vi "Configure Sampling.vi"(0 "VISA resource in":refnum<visa-resource-name>, 1 "sample period [s] (-1: use EXT trig as source)":dbl=-1.0 format="%#_6p", 2 "apperture [s] (1.4us)":dbl=1.4e-06 format="%#_6p", 3 "LEVEL trigger":T1 caption="Cluster", 4 "EXT OUT signal (APER)":T2, 5 "error in":errorcluster, 6 "range [V] (10V)":dbl=10.0, 7 "samples count (100)":i32=100, 10 "sampling mode (DCV)":T3, 11 "delay [s]":dbl=1e-07, 12 "stream mode (False)":bool, 13 "first sample (AUTO)":T4) -> (14 "VISA resource name out":refnum<visa-resource-name>, 19 "error out":errorcluster)   [LabVIEW 2018, in "3458A Virtual Digitizer.lvlib" / "3458A Digitizing Low Levels.lvlib"]
doc: "This VI configures DMM for digitizing of sequence of samples. It will enable the mode (DCV, DSDC, DSAC), then it will decide sample clocking source (TIMER or EXT), decides format of memory/data transfer based on aperture (SINT, DINT) and puts the meter in TARM HOLD mode so it is ready to start when DMM is armed. When stream mode is enabled it disables memory so the data will be sent directly to the controller. Frist sample input specifies what is used as trigger source. Default is AUTO. For stream mode SYN mode is convenient because it will trigger when controller is ready to receive.\n\nNote: Reentrant VI so it can be executed in parallel for multiple 3458A sessions."
uses:
  3458A Digitizing Low Levels.lvlib
  First Sample Trigger.ctl
  Sampling Mode.ctl
  EXT OUT mode.ctl
  Level Setup.ctl
  3458A Basic Driver/3458A Basic Driver.lvlib
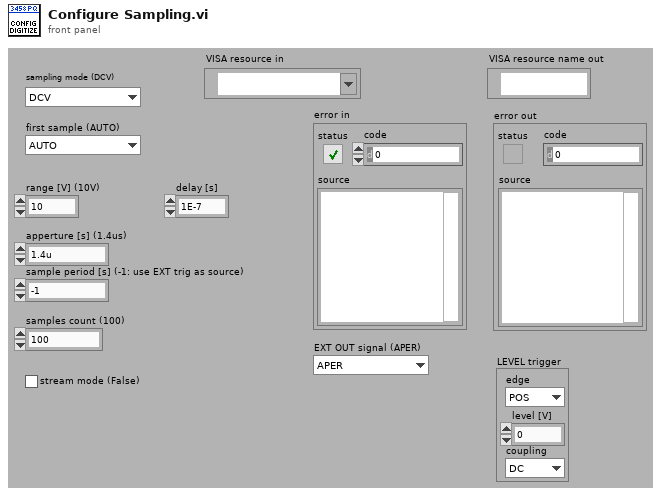
[diagram p1: front panel]
types:
  T1 = typedef "3458A Virtual Digitizer.lvlib/3458A Digitizing Low Levels.lvlib/Level Setup.ctl" = cluster{"edge":enum16{"POS", "NEG"}, "level [V]":dbl, "coupling":enum16{"DC", "AC"}}
  T2 = typedef "3458A Virtual Digitizer.lvlib/3458A Digitizing Low Levels.lvlib/EXT OUT mode.ctl" = enum16{"APER", "ICOMP"}
  T3 = typedef "3458A Virtual Digitizer.lvlib/3458A Digitizing Low Levels.lvlib/Sampling Mode.ctl" = enum16{"DCV", "DSDC", "DSAC"}
  T4 = typedef "3458A Virtual Digitizer.lvlib/3458A Digitizing Low Levels.lvlib/First Sample Trigger.ctl" = enum16{"AUTO", "EXT", "SYN", "SGL", "HOLD", "LEVEL"}
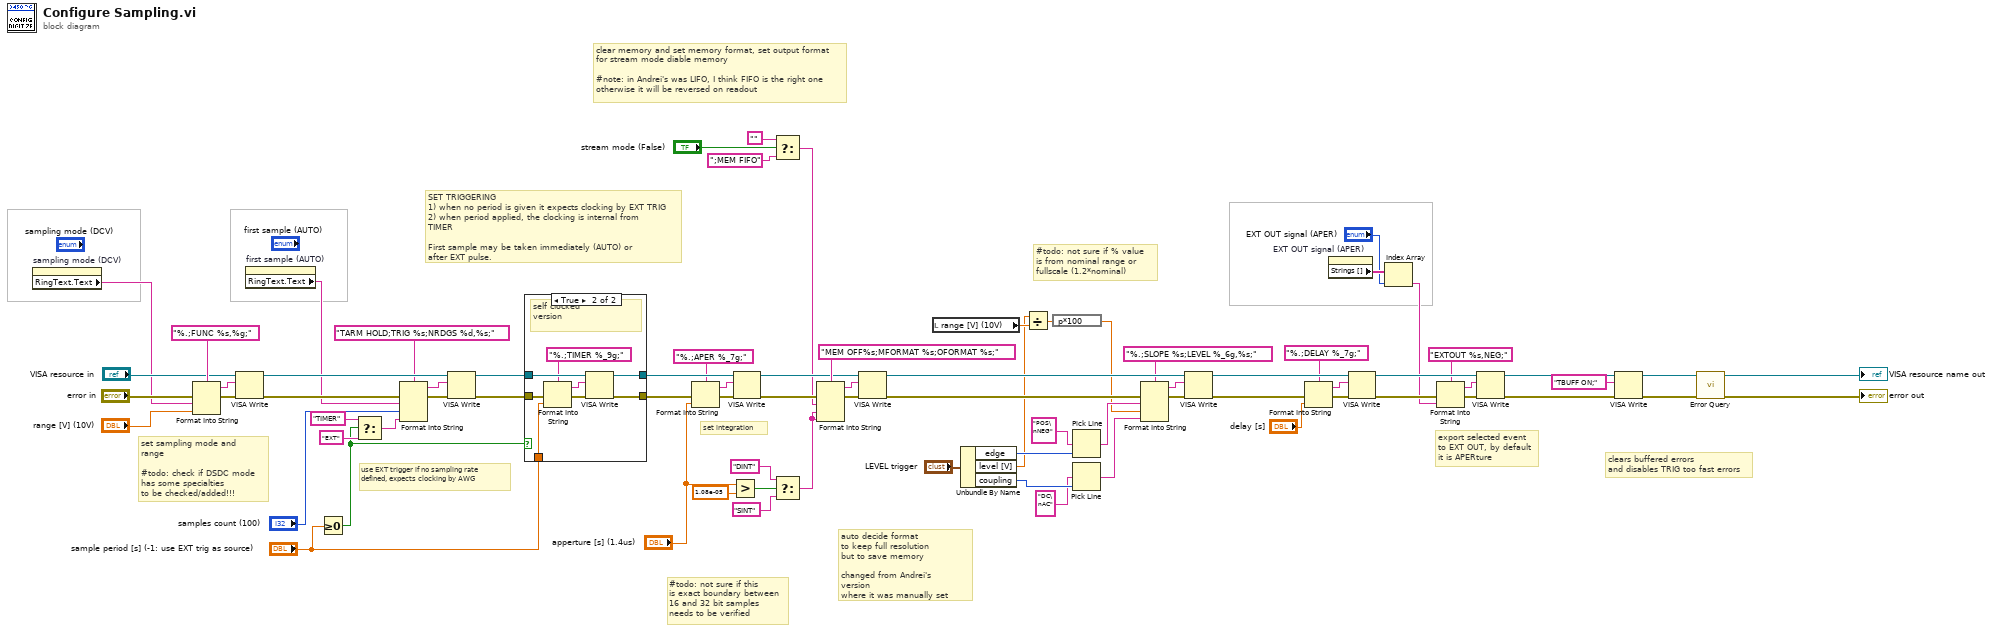
[diagram p0: block diagram]
diagram:
  # "#todo: not sure if % value\nis from nominal range or \nfullscale (1.2*nominal)"
  # "clears buffered errors\nand disables TRIG too fast errors"
  # "export selected event\nto EXT OUT, by default\nit is APERture"
  # "#todo: not sure if this\nis exact boundary between\n16 and 32 bit samples\nneeds to be verified"
  # "clear memory and set memory format, set output format\nfor stream mode diable memory\n\n#note: in Andrei's was LIFO, I think FIFO is the right one\notherwise it will be reversed on readout"
  # "auto decide format\nto keep full resolution\nbut to save memory\n\nchanged from Andrei's version\nwhere it was manually set"
  # "set integration"
  # "use EXT trigger if no sampling rate\ndefined, expects clocking by AWG"
  # "SET TRIGGERING\n1) when no period is given it expects clocking by EXT TRIG\n2) when period applied, the clocking is internal from TIMER\n\nFirst sample may be taken immediately (AUTO) or \nafter EXT pulse."
  # "set sampling mode and range\n\n#todo: check if DSDC mode has some specialties\nto be checked/added!!!"
  n1 = property on="sampling mode (DCV)" class="Enum (strict)"() -> ("RingText.Text"=w42:string)  [unwired: 2 in, 2 out]
  n2 = Format Into String(format string="%.;FUNC %s,%g;" ("write buffer"), error in="error in", w42, "range [V] (10V)") -> (resulting string=w77:string, error out=w78:errorcluster)  [unwired: 1 in]
  n3 = VISA Write(VISA resource name="VISA resource in", write buffer=w77, error in (no error)=w78) -> (VISA resource name out=w75:refnum<visa-resource-name>, error out=w67:errorcluster)  [unwired: 1 out]
  n4 = property on="first sample (AUTO)" class="Enum (strict)"() -> ("RingText.Text"=w46:string)  [unwired: 2 in, 2 out]
  n5 = Greater Or Equal To 0?(x="sample period [s] (-1: use EXT trig as source)") -> (x >= 0?=w63:bool)
  n6 = Select(t="TIMER" ("multi-line string"), s=w63, f="EXT" ("multi-line string")) -> (s? t:f=w68:string)
  n7 = Format Into String(format string="TARM HOLD;TRIG %s;NRDGS %d,%s;", error in=w67, w46, "samples count (100)", w68) -> (resulting string=w72:string, error out=w74:errorcluster)  [unwired: 1 in]
  n8 = VISA Write(VISA resource name=w75, write buffer=w72, error in (no error)=w74) -> (VISA resource name out=w65:refnum<visa-resource-name>, error out=w66:errorcluster)  [unwired: 1 out]
  n9 = case shown="True" w63 {
    tunnel: w66 -> [w79 w88]
    tunnel: w65 -> [w80 w86]
    tunnel: "sample period [s] (-1: use EXT trig as source)" -> [_ w84]
    tunnel: [w79 w83] -> w60
    tunnel: [w80 w82] -> w59
    frame False {
      # "EXT clocked"
    }
    frame True {
      # "self clocked\nversion"
      n10 = Format Into String(format string="%.;TIMER %_9g;" ("write buffer"), error in=w88, w84) -> (resulting string=w81:string, error out=w87:errorcluster)  [unwired: 1 in]
      n11 = VISA Write(VISA resource name=w86, write buffer=w81, error in (no error)=w87) -> (VISA resource name out=w82:refnum<visa-resource-name>, error out=w83:errorcluster)  [unwired: 1 out]
    }
  }
  n12 = Format Into String(format string="%.;APER %_7g;", error in=w60, "apperture [s] (1.4us)") -> (resulting string=w62:string, error out=w61:errorcluster)  [unwired: 1 in]
  n13 = Greater?(x="apperture [s] (1.4us)", y=1.08e-05) -> (0:w50:bool)
  n14 = VISA Write(VISA resource name=w59, write buffer=w62, error in (no error)=w61) -> (VISA resource name out=w55:refnum<visa-resource-name>, error out=w54:errorcluster)  [unwired: 1 out]
  n15 = Select(t="", s="stream mode (False)", f=";MEM FIFO" ("write buffer")) -> (s? t:f=w35:string)
  n16 = Select(t="DINT" ("format string"), s=w50, f="SINT" ("format string")) -> (s? t:f=w47:string)
  n17 = Format Into String(format string="MEM OFF%s;MFORMAT %s;OFORMAT %s;" ("write buffer"), error in=w54, w35, w47, w47) -> (resulting string=w57:string, error out=w58:errorcluster)  [unwired: 1 in]
  n18 = VISA Write(VISA resource name=w55, write buffer=w57, error in (no error)=w58) -> (VISA resource name out=w20:refnum<visa-resource-name>, error out=w17:errorcluster)  [unwired: 1 out]
  n19 = local read "range [V] (10V)"() -> (w8:dbl)
  n20 = Unbundle By Name("LEVEL trigger") -> ("edge"=w14:enum16{"POS", "NEG"}, "level [V]"=w7:dbl, "coupling"=w12:enum16{"DC", "AC"})
  n21 = Divide(x=w7, y=w8) -> (x/y=w6:dbl)
  n22 = expression code="p*100"(w6) -> (w5:dbl)
  n23 = Pick Line(multi-line string="POS\nNEG" ("string (\"\")"), line index=w14) -> (output string=w13:string)  [unwired: 1 in]
  n24 = Pick Line(multi-line string="DC\nAC" ("string (\"\")"), line index=w12) -> (output string=w11:string)  [unwired: 1 in]
  n25 = Format Into String(format string="%.;SLOPE %s;LEVEL %_6g,%s;" ("write buffer"), error in=w17, w13, w5, w11) -> (resulting string=w16:string, error out=w18:errorcluster)  [unwired: 1 in]
  n26 = VISA Write(VISA resource name=w20, write buffer=w16, error in (no error)=w18) -> (VISA resource name out=w34:refnum<visa-resource-name>, error out=w31:errorcluster)  [unwired: 1 out]
  n27 = Format Into String(format string="%.;DELAY %_7g;" ("write buffer"), error in=w31, "delay [s]") -> (resulting string=w32:string, error out=w33:errorcluster)  [unwired: 1 in]
  n28 = property on="EXT OUT signal (APER)" class="Enum (strict)"() -> ("Strings []"=w23:string[])  [unwired: 2 in, 2 out]
  n29 = VISA Write(VISA resource name=w34, write buffer=w32, error in (no error)=w33) -> (VISA resource name out=w26:refnum<visa-resource-name>, error out=w28:errorcluster)  [unwired: 1 out]
  n30 = Index Array(array=w23, index="EXT OUT signal (APER)") -> (element=w21:string)
  n31 = Format Into String(format string="EXTOUT %s,NEG;" ("write buffer"), error in=w28, w21) -> (resulting string=w25:string, error out=w27:errorcluster)  [unwired: 1 in]
  n32 = VISA Write(VISA resource name=w26, write buffer=w25, error in (no error)=w27) -> (VISA resource name out=w40:refnum<visa-resource-name>, error out=w41:errorcluster)  [unwired: 1 out]
  n33 = VISA Write(VISA resource name=w40, write buffer="TBUFF ON;", error in (no error)=w41) -> (VISA resource name out=w3:refnum<visa-resource-name>, error out=w4:errorcluster)  [unwired: 1 out]
  n34 = call "Error Query.vi"("error in (no error)"=w4, "VISA resource name"=w3) -> ("error out"=→"error out":errorcluster, "VISA resource name out"=→"VISA resource name out":refnum<visa-resource-name>)  [unwired: 6 in, 2 out]
